vi "_Calculate Check Sum.vi"(1 "Stream":string) -> (0 "Checksum":u32)   [LabVIEW 2015]
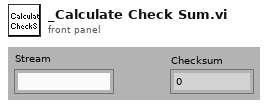
[diagram p1: front panel]
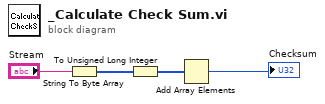
[diagram p0: block diagram]
diagram:
  n1 = String To Byte Array(string="Stream") -> (unsigned byte array=w4:u8[])
  n2 = To Unsigned Long Integer(number=w4) -> (unsigned 32bit integer=w2:u32[])
  n3 = Add Array Elements(numeric array=w2) -> (sum=→"Checksum":u32)
